vi "AD Remove Disabled.vi"(3 "Items In":string[](array[string])) -> (0 "Item(s) Removed":bool, 1 "Items Out":string[](array[string]))   [LabVIEW 2019]
uses:
  2020 Robot/Framework/Robot Global Data.vi
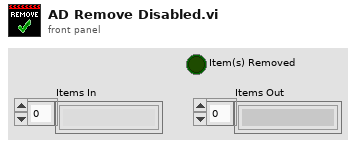
[diagram p1: front panel]
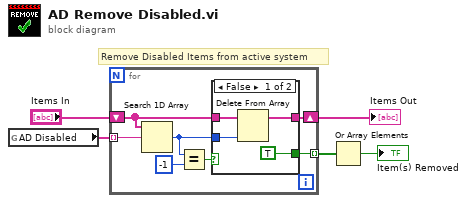
[diagram p0: block diagram]
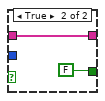
[diagram p2: hidden frame]
diagram:
  # "Remove Disabled Items from active system"
  n1 = global read "Robot Global Data.vi" "AD Disabled"() -> (w3:string[])
  n2 = for {
    tunnel: w3 -> [w11] mode=indexing
    shift-right: [w9] -> w5
    shift-left: "Items In" -> [w7]
    tunnel: [w6] -> w2 mode=indexing
    n3 = Search 1D Array(1D array=w7, element=w11) -> (index of element=w8:i32)  [unwired: 1 in]
    n4 = Equal?(x=w8, y=-1) -> (x = y?=w10:bool)
    n5 = case shown="False" w10 {
      tunnel: w7 -> [w16 w18]
      tunnel: [w15 w18] -> w9
      tunnel: w8 -> [w14 _]
      tunnel: [TRUE FALSE] -> w6
      frame False {
        n6 = Delete From Array(array=w16, index=w14) -> (array with subset deleted=w15:string[])  [unwired: 1 in, 1 out]
      }
      frame True {
      }
    }
  }
  "Items Out" <- w5
  n7 = Or Array Elements(Boolean array=w2) -> (logical OR=→"Item(s) Removed":bool)
